vi "Set Syringe Volume.vi"(7 "Volume Units (0:ml)":u16(ring)=2 items=["microliters", "nanoliters", "milliliters"], 8 "error in (no error)":errorcluster, 9 "Query?":bool, 10 "Syringe volume":i32=1 min=0 max=999 step=1, 11 "VISA resource name":refnum<visa-resource-name>) -> (0 "error out":errorcluster, 2 "Output syringe volume":string, 3 "VISA resource name out":refnum<visa-resource-name>)   [LabVIEW 2016]
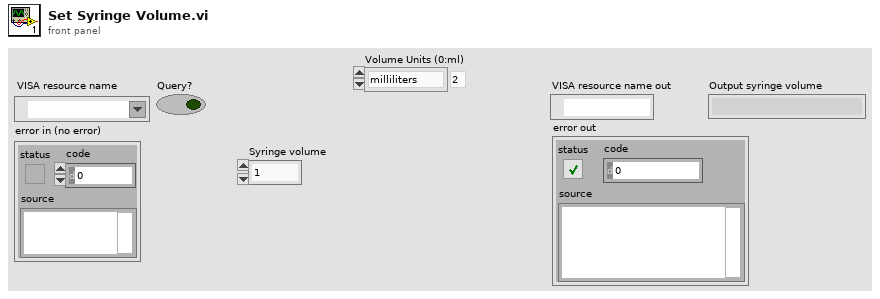
[diagram p1: front panel]
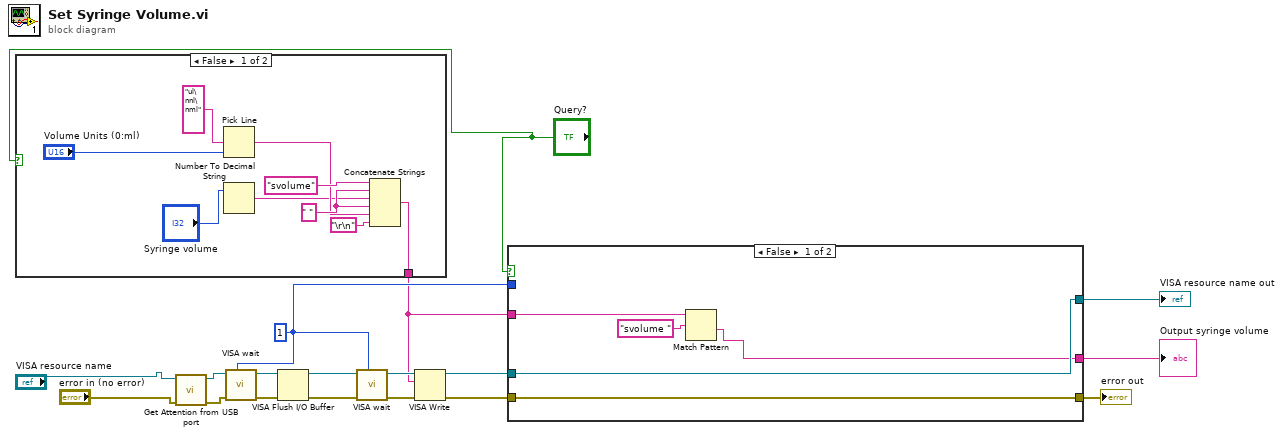
[diagram p0: block diagram]
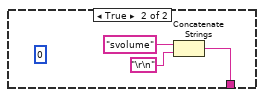
[diagram p2: hidden frame]
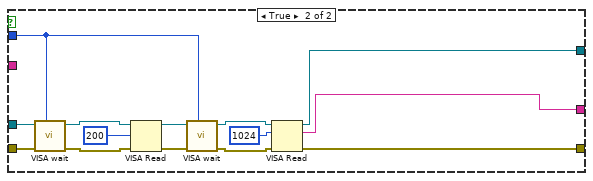
[diagram p3: hidden frame]
diagram:
  w8 = u32 1 ("milliseconds to wait")
  n1 = case shown="False" "Query?" {
    tunnel: [w20 w28] -> w6
    frame False {
      w24 = " " ("string")
      n2 = Pick Line(multi-line string="ul\nnl\nml", line index="Volume Units (0:ml)") -> (output string=w23:string)  [unwired: 1 in]
      n3 = Number To Decimal String(number="Syringe volume") -> (decimal integer string=w21:string)  [unwired: 1 in]
      n4 = Concatenate Strings("svolume" ("string"), w24, w21, w24, w23, "\r\n") -> (w20:string)
    }
    frame True {
      (unwired) 0 ("Volume")
      n5 = Concatenate Strings("svolume" ("string"), "\r\n") -> (w28:string)
    }
  }
  n6 = call "Get Attention from USB port.vi"("error in (no error)"="error in (no error)", "VISA resource name"="VISA resource name") -> ("error out"=w3:errorcluster, "VISA resource name out"=w4:refnum<visa-resource-name>)  [unwired: 8 in]
  n7 = call <userlib>:"VISA wait.vi"("VISA resource name"=w4, "error in (no error)"=w3, "milliseconds to wait"=w8) -> ("VISA resource name out"=w17:refnum<visa-resource-name>, "error out"=w18:errorcluster)  [unwired: 6 in]
  n8 = VISA Flush I/O Buffer(VISA resource name=w17, error in (no error)=w18) -> (VISA resource name out=w16:refnum<visa-resource-name>, error out=w15:errorcluster)  [unwired: 1 in]
  n9 = call <userlib>:"VISA wait.vi"("VISA resource name"=w16, "error in (no error)"=w15, "milliseconds to wait"=w8) -> ("VISA resource name out"=w13:refnum<visa-resource-name>, "error out"=w14:errorcluster)  [unwired: 6 in]
  n10 = VISA Write(VISA resource name=w13, write buffer=w6, error in (no error)=w14) -> (VISA resource name out=w12:refnum<visa-resource-name>, error out=w11:errorcluster)  [unwired: 1 out]
  n11 = case shown="False" "Query?" {
    tunnel: w12 -> [w35 w49]
    tunnel: w11 -> [w34 w48]
    tunnel: [w35 w41] -> w10
    tunnel: [w34 w40] -> w9
    tunnel: w8 -> [_ w39]
    tunnel: [w32 w36] -> w7
    tunnel: w6 -> [w33 _]
    frame False {
      n12 = Match Pattern(string=w33, regular expression="svolume ") -> (after substring=w32:string)  [unwired: 1 in, 3 out]
    }
    frame True {
      n13 = call <userlib>:"VISA wait.vi"("VISA resource name"=w49, "error in (no error)"=w48, "milliseconds to wait"=w39) -> ("VISA resource name out"=w46:refnum<visa-resource-name>, "error out"=w47:errorcluster)  [unwired: 6 in]
      n14 = VISA Read(VISA resource name=w46, byte count=u32 200, error in (no error)=w47) -> (VISA resource name out=w45:refnum<visa-resource-name>, error out=w44:errorcluster)  [unwired: 2 out]
      n15 = call <userlib>:"VISA wait.vi"("VISA resource name"=w45, "error in (no error)"=w44, "milliseconds to wait"=w39) -> ("VISA resource name out"=w42:refnum<visa-resource-name>, "error out"=w43:errorcluster)  [unwired: 6 in]
      n16 = VISA Read(VISA resource name=w42, byte count=u32 1024, error in (no error)=w43) -> (VISA resource name out=w41:refnum<visa-resource-name>, read buffer=w36:string, error out=w40:errorcluster)  [unwired: 1 out]
    }
  }
  "VISA resource name out" <- w10
  "error out" <- w9
  "Output syringe volume" <- w7
